vi "Error Handler - Message Handling Loop.vi"(8 "error in (no error)":T1 caption="entrée d'erreur (pas d'erreur)", 10 "Erreurs à ignorer (exécution)":i32[](array[numeric]), 11 "File d'attente de messages":refnum<queue>) -> (0 "erreur en entrée dup.":T1, 3 "File d'attente de message dup.":refnum<queue>)   [LabVIEW 2020]
doc: "Gère une erreur qui a eu lieu dans la boucle de gestion de messages en l'ignorant ou en générant un message \"Exit\"."
uses:
  Message Queue/Message Cluster.ctl
  Message Queue/Message Queue.lvlib
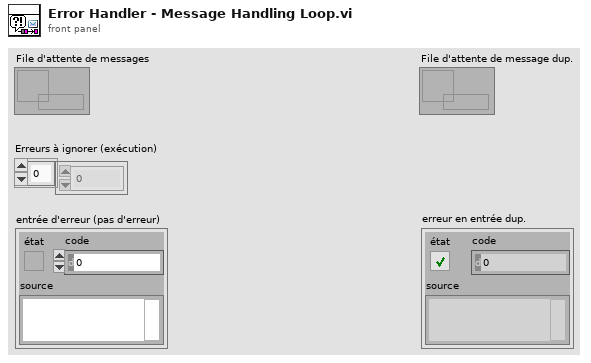
[diagram p1: front panel]
types:
  T1 = cluster{"état":bool, "code":i32, "source":string}
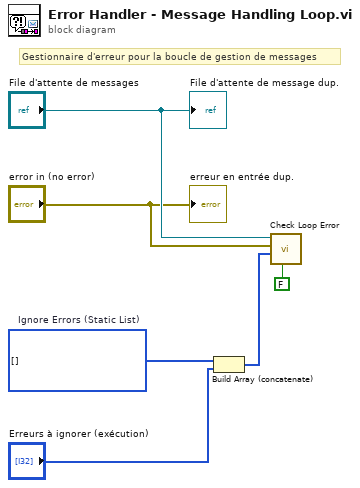
[diagram p0: block diagram]
diagram:
  w5 = i32[] []  # Ignore Errors (Static List)
  # "Gestionnaire d'erreur pour la boucle de gestion de messages"
  n1 = Build Array (concatenate)(w5, "Erreurs à ignorer (exécution)") -> (w4:i32[])
  n2 = call "Check Loop Error.vi"("Quitter en cas d'erreur ? (F)"=FALSE ("Exit on Error? (F)"), "Ignorer les erreurs"=w4, "erreur à traiter"="error in (no error)", "File d'attente de messages"="File d'attente de messages") -> ()  [unwired: 6 in, 2 out]
  "File d'attente de message dup." <- "File d'attente de messages"
  "erreur en entrée dup." <- "error in (no error)"
